vi "ExEventOpen.vi"(0 "error in (no error)":errorcluster) -> (1 "Major Time":u32, 2 "Minor Time":u32, 4 "error out":errorcluster)   [LabVIEW 2015]
uses:
  BC637PCI.dll
panel:
  out "Nano":u16
  out "Return":i32
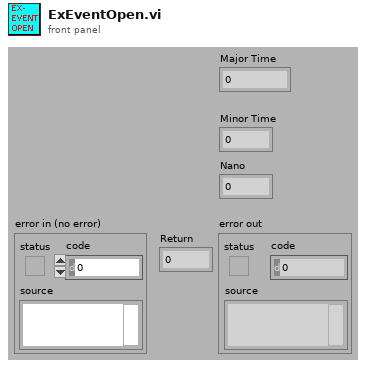
[diagram p1: front panel]
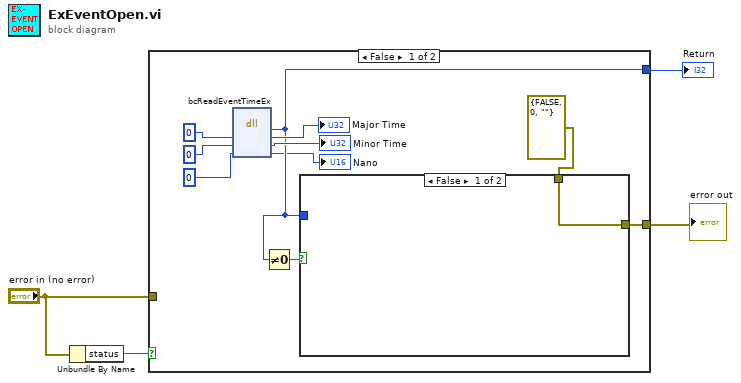
[diagram p0: block diagram]
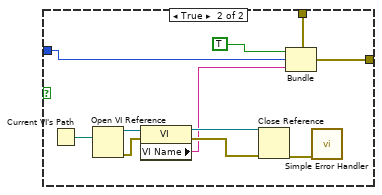
[diagram p2: hidden frame]
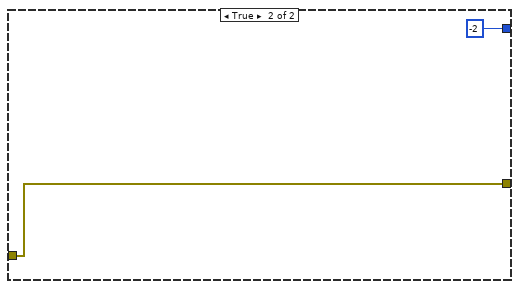
[diagram p3: hidden frame]
diagram:
  n1 = Unbundle By Name("error in (no error)") -> ("status"=w1:bool)
  n2 = case shown="False" w1 {
    tunnel: [w6 -2] -> w4
    tunnel: "error in (no error)" -> [_ w27]
    tunnel: [w9 w27] -> w3
    frame False {
      n3 = dll-call lib="C:/GSCS 2.0/GSCS/Systems/SIcamera_Control/GPS_Drivers/BC637PCI.dll" fn="bcReadEventTimeEx"("maj"=u32 0, "min"=u32 0, "nano"=u16 0) -> ("return type"=w6:i32, "maj"=→"Major Time":u32, "min"=→"Minor Time":u32, "nano"=→"Nano":u16)  [unwired: 3 in, 2 out]
      n4 = Not Equal To 0?(x=w6) -> (x != 0?=w10:bool)
      n5 = case shown="False" w10 {
        tunnel: w6 -> [_ w19]
        tunnel: [w15 w17] -> w9
        tunnel: errorcluster {FALSE, 0, ""} -> [w15 w16]
        frame False {
        }
        frame True {
          n6 = Current VI's Path() -> (path=w26:path)
          n7 = Open VI Reference(vi path=w26) -> (vi reference=w24:refnum<vi>, error out=w25:errorcluster)  [unwired: 5 in]
          n8 = property class="VI"(reference=w24, error in=w25) -> (reference out=w23:refnum<vi>, error out=w22:errorcluster, "VI Name"=w18:string)
          n9 = Close Reference(reference=w23, error in (no error)=w22) -> (error out=w21:errorcluster)
          n10 = Bundle(cluster=w16, TRUE, w19, w18) -> (w17:errorcluster)
          n11 = call <vilib>:"Simple Error Handler.vi"("error in (no error)"=w21) -> ()  [unwired: 4 in, 5 out]
        }
      }
    }
    frame True {
    }
  }
  "Return" <- w4
  "error out" <- w3
